vi "Histogram Main.vi"() -> ()   [LabVIEW 2015]
uses:
  Consumer Message.ctl
  <vilib>/ErrorRing/Error Ring.xnode
panel:
  in  "signal":u16(ring) items=["uniform white", "uniform+uniform", "Gaussian white", "sine", "square"]
  out "Consumer Shutdown?":bool
  out "State to Execute":string
  out "High Priority?":bool
  out "Backlog":u8(slide) scale=0.0..100.0
  out "Processed Value":i32
  in  "High Priority Message":bool
  in  "Normal Priority Message":bool
  in  "Stop":bool
  # "Number of enqueued messages waiting to be processed"
  # "Current data being processed in consumer loop"
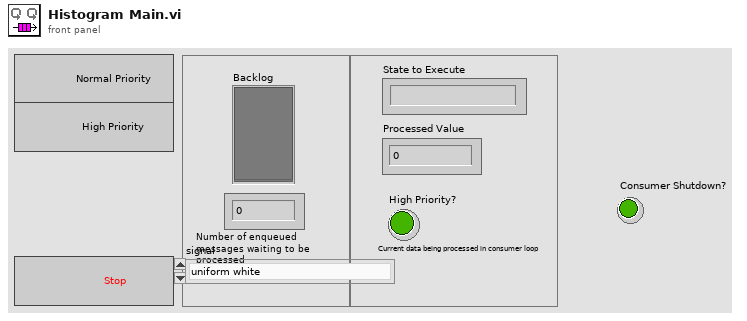
[diagram p1: front panel]
types:
  T1 = typedef "Consumer Message.ctl" = cluster{"Consumer State":string, "Boolean Data":bool, "Numeric Data":i32, "Signal":dbl[], "Error":errorcluster}
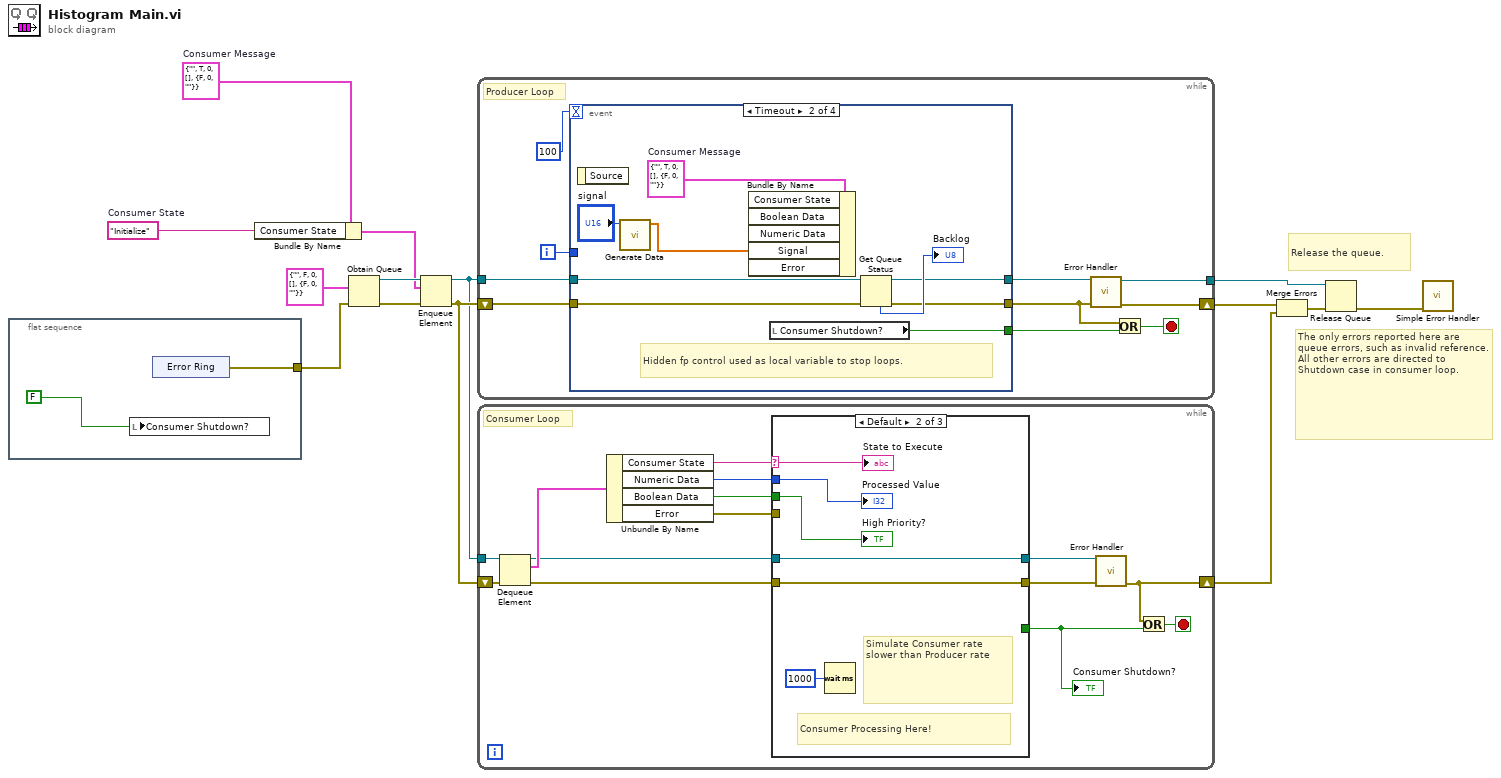
[diagram p0: block diagram]
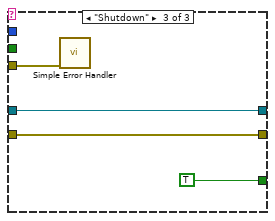
[diagram p3: hidden frame]
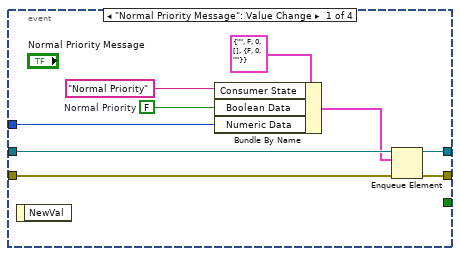
[diagram p4: hidden frame]
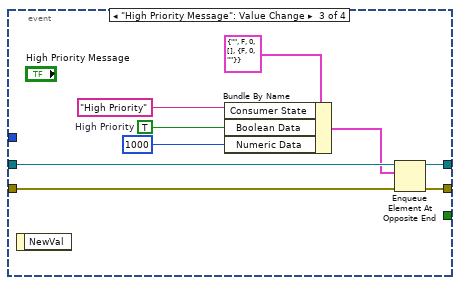
[diagram p5: hidden frame]
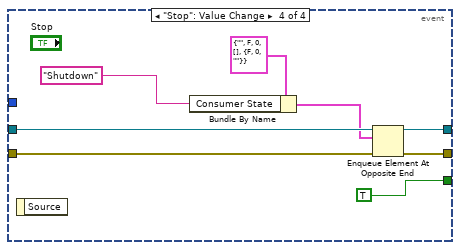
[diagram p6: hidden frame]
diagram:
  w6 = "Initialize"  # Consumer State
  w8 = T1 {"Consumer State"="", "Boolean Data"=TRUE, "Numeric Data"=0, "Signal"=[], "Error"={"status"=FALSE, "code"=0, "source"=""}}  # Consumer Message
  # "Release the queue."
  # "The only errors reported here are queue errors, such as invalid reference.  All other errors are directed to Shutdown case in consumer loop."
  n1 = flat-sequence {
    tunnel: [w15] -> w9
    frame #0 {
      n2 = local write "Consumer Shutdown?"(FALSE ("Stop Loops (local)")) -> ()
      n3 = xnode "Error Ring"() -> ("error out"=w15:errorcluster)
    }
  }
  n4 = Bundle By Name(cluster=w8, "Consumer State"=w6) -> (w7:T1)
  n5 = Obtain Queue(element data type=T1 {"Consumer State"="", "Boolean Data"=FALSE, "Numeric Data"=0, "Signal"=[], "Error"={"status"=FALSE, "code"=0, "source"=""}}, error in (no error)=w9) -> (queue out=w11:refnum<queue>, error out=w14:errorcluster)  [unwired: 3 in, 1 out]
  n6 = Enqueue Element(queue=w11, element=w7, error in (no error)=w14) -> (queue out=w10:refnum<queue>, error out=w12:errorcluster)  [unwired: 1 in, 1 out]
  n7 = while {
    tunnel: w10 -> [w27]
    shift-right: [w19] -> w5
    shift-left: w12 -> [w26]
    tunnel: [w18] -> w1
    i -> [w25]
    stop <- w21 stop-if-true
    # "Producer Loop"
    n8 = event shown="[1] Timeout" {
      selector: _ -> [_ _ _ _]
      dyn-events: _ -> [_ _ _ _]
      timeout: 100 -> [_ _ _ _]
      tunnel: w27 -> [w36 w43 w53 w62]
      tunnel: w26 -> [w34 w42 w52 w60]
      tunnel: [w35 w41 w54 w59] -> w20
      tunnel: [_ w45 _ TRUE] -> w22
      tunnel: w25 -> [w33 _ _ _]
      tunnel: [w29 w40 w48 w58] -> w24
      event "Normal Priority Message": Value Change {
        w30 = FALSE  # Normal Priority
        n9 = event-data() -> ()  [unwired: 1 in, 1 out]
        n10 = Bundle By Name(cluster=T1 {"Consumer State"="", "Boolean Data"=FALSE, "Numeric Data"=0, "Signal"=[], "Error"={"status"=FALSE, "code"=0, "source"=""}}, "Consumer State"="Normal Priority" ("String Data"), "Boolean Data"=w30, "Numeric Data"=w33) -> (w32:T1)
        n11 = Enqueue Element(queue=w36, element=w32, error in (no error)=w34) -> (queue out=w29:refnum<queue>, error out=w35:errorcluster)  [unwired: 1 in, 1 out]
      }
      event Timeout {
        w39 = T1 {"Consumer State"="", "Boolean Data"=TRUE, "Numeric Data"=0, "Signal"=[], "Error"={"status"=FALSE, "code"=0, "source"=""}}  # Consumer Message
        # "Hidden fp control used as local variable to stop loops."
        n12 = event-data() -> ()  [unwired: 1 in, 1 out]
        n13 = call "Generate Data.vi"("signal"="signal") -> ("Y"=w38:dbl[])  [unwired: 9 in, 1 out]
        n14 = Bundle By Name(cluster=w39, "Signal"=w38) -> ()  [unwired: 4 in, 1 out]
        n15 = local read "Consumer Shutdown?"() -> (w45:bool)
        n16 = Get Queue Status(queue=w43, error in (no error)=w42) -> (queue out=w40:refnum<queue>, error out=w41:errorcluster, # elements in queue=→"Backlog":i32)  [unwired: 1 in, 5 out]
      }
      event "High Priority Message": Value Change {
        w47 = TRUE  # High Priority
        n17 = event-data() -> ()  [unwired: 1 in, 1 out]
        n18 = Bundle By Name(cluster=T1 {"Consumer State"="", "Boolean Data"=FALSE, "Numeric Data"=0, "Signal"=[], "Error"={"status"=FALSE, "code"=0, "source"=""}}, "Consumer State"="High Priority" ("String Data"), "Boolean Data"=w47, "Numeric Data"=1000) -> (w50:T1)
        n19 = Enqueue Element At Opposite End(queue=w53, element=w50, error in (no error)=w52) -> (queue out=w48:refnum<queue>, error out=w54:errorcluster)  [unwired: 1 in, 1 out]
      }
      event "Stop": Value Change {
        n20 = event-data() -> ()  [unwired: 1 in, 1 out]
        n21 = Bundle By Name(cluster=T1 {"Consumer State"="", "Boolean Data"=FALSE, "Numeric Data"=0, "Signal"=[], "Error"={"status"=FALSE, "code"=0, "source"=""}}, "Consumer State"="Shutdown") -> (w55:T1)
        n22 = Enqueue Element At Opposite End(queue=w62, element=w55, error in (no error)=w60) -> (queue out=w58:refnum<queue>, error out=w59:errorcluster)  [unwired: 1 in, 1 out]
      }
    }
    n23 = call "Error Handler.vi"("error in"=w20, "queue in"=w24) -> ("error out"=w19:errorcluster, "queue out"=w18:refnum<queue>)  [unwired: 8 in]
    n24 = Or(x=w20, y=w22) -> (x .or. y?=w21:bool)
  }
  n25 = while {
    tunnel: w10 -> [w76]
    shift-right: [w65] -> w4
    shift-left: w12 -> [w75]
    stop <- w66 stop-if-true
    # "Consumer Loop"
    n26 = Dequeue Element(queue=w76, error in (no error)=w75) -> (queue out=w64:refnum<queue>, element=w74:T1, error out=w63:errorcluster)  [unwired: 1 in, 1 out]
    n27 = Unbundle By Name(w74) -> ("Consumer State"=w73:string, "Numeric Data"=w72:i32, "Boolean Data"=w71:bool, "Error"=w68:errorcluster)
    n28 = case shown="Default" w73 {
      selector: w73 -> [_ w81 _]
      tunnel: [_ _ TRUE] -> w67
      tunnel: w63 -> [w77 w79 w85]
      tunnel: [w77 w79 w85] -> w70
      tunnel: w72 -> [_ w84 _]
      tunnel: w71 -> [_ w83 _]
      tunnel: w64 -> [w78 w82 w86]
      tunnel: [w78 w82 w86] -> w69
      tunnel: w68 -> [_ _ w87]
      frame "Initialize" {
      }
      frame Default {
        # "Simulate Consumer rate slower than Producer rate"
        # "Consumer Processing Here!"
        n29 = Wait (ms)(milliseconds to wait=u32 1000) -> ()  [unwired: 1 out]
        "Processed Value" <- w84
        "High Priority?" <- w83
        "State to Execute" <- w81
      }
      frame "Shutdown" {
        n30 = call <vilib>:"Simple Error Handler.vi"("error in (no error)"=w87) -> ()  [unwired: 4 in, 5 out]
      }
    }
    "Consumer Shutdown?" <- w67
    n31 = call "Error Handler.vi"("error in"=w70, "queue in"=w69) -> ("error out"=w65:errorcluster)  [unwired: 8 in, 1 out]
    n32 = Or(x=w65, y=w67) -> (x .or. y?=w66:bool)
  }
  n33 = Merge Errors(w5, w4) -> (w3:errorcluster)
  n34 = Release Queue(queue=w1, error in (no error)=w3) -> (error out=w2:errorcluster)  [unwired: 1 in, 2 out]
  n35 = call <vilib>:"Simple Error Handler.vi"("error in (no error)"=w2) -> ()  [unwired: 4 in, 5 out]
